vi "Convert .NET Exception.vi"(2 "error in (no error)":errorcluster, 3 "Operation":string, 4 "Report Ref In":T1) -> (0 "error out":errorcluster, 1 "Report Ref Out":T1)   [LabVIEW 2013, in "XCel Report Engine.lvlib"]
doc: "Processes errors generated by .NET constructor and invoke nodes used by XCelReportEngine wrapper VIs.\n\nThis private helper preserves the LabVIEW error cluster and provides a central location for translating .NET exceptions into consistent XCelReportEngine error information.\n\nIt is intended for internal use by the report engine library and should not be called directly by application code."
uses:
  XCel Report Engine.lvlib
  Controls/Report Ref.ctl
  C:/Users/m.santucci/Documents/ChatGPT/LV_REPORT_ENGINE/LV/DotNet/XCelReportEngine.dll
  LV/DotNet/XCelReportEngine.dll
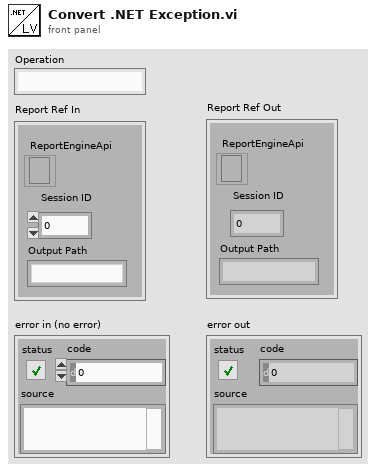
[diagram p1: front panel]
types:
  T1 = typedef "XCel Report Engine.lvlib/Report Ref.ctl" = cluster{"Session ID":i32, "Output Path":string, "ReportEngineApi":refnum<k24>}
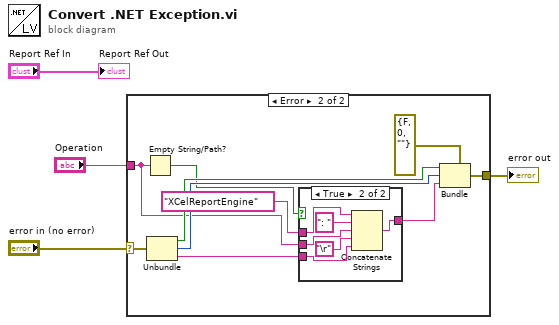
[diagram p0: block diagram]
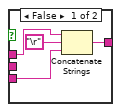
[diagram p3: hidden frame]
diagram:
  n1 = case shown="Error" "error in (no error)" {
    selector: "error in (no error)" -> [w5 w14]
    tunnel: [w5 w6] -> w2
    tunnel: "Operation" -> [_ w9]
    frame No Error {
    }
    frame Error {
      n2 = Empty String/Path?(string/path=w9) -> (empty?=w11:bool)
      n3 = Unbundle(w14) -> ("status"=w13:bool, "code"=w12:i32, "source"=w7:string)
      n4 = case shown="True" w11 {
        tunnel: "XCelReportEngine" -> [w19 w25]
        tunnel: w9 -> [_ w24]
        tunnel: [w18 w21] -> w8
        tunnel: w7 -> [w17 w20]
        frame False {
          n5 = Concatenate Strings(w19, "\r", w17) -> (w18:string)
        }
        frame True {
          n6 = Concatenate Strings(w25, ": " ("string"), w24, "\r", w20) -> (w21:string)
        }
      }
      n7 = Bundle(cluster=errorcluster {"status"=FALSE, "code"=0, "source"=""} ("error IO"), "status"=w13, "code"=w12, "source"=w8) -> (w6:errorcluster)
    }
  }
  "error out" <- w2
  "Report Ref Out" <- "Report Ref In"
